vi "SendBuffReceiveCS (SubVI).vi"(8 "error in (no error)":errorcluster, 9 "Array in":u8[](array[numeric]), 10 "ExpectedCheckSum":string, 11 "VISA Refnum in":refnum<visa-resource-name>) -> (0 "error out":errorcluster, 1 "CorrectCheckSum?":bool, 2 "Timeout?":bool, 3 "VISA Refnum out":refnum<visa-resource-name>)   [LabVIEW 2017]
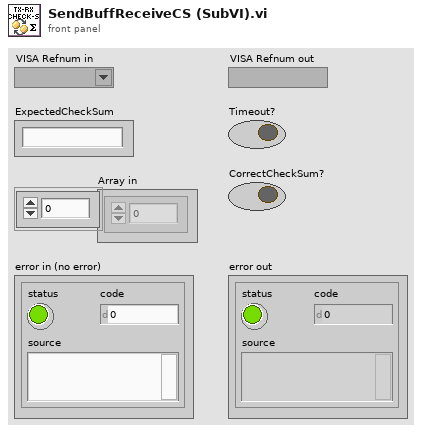
[diagram p1: front panel]
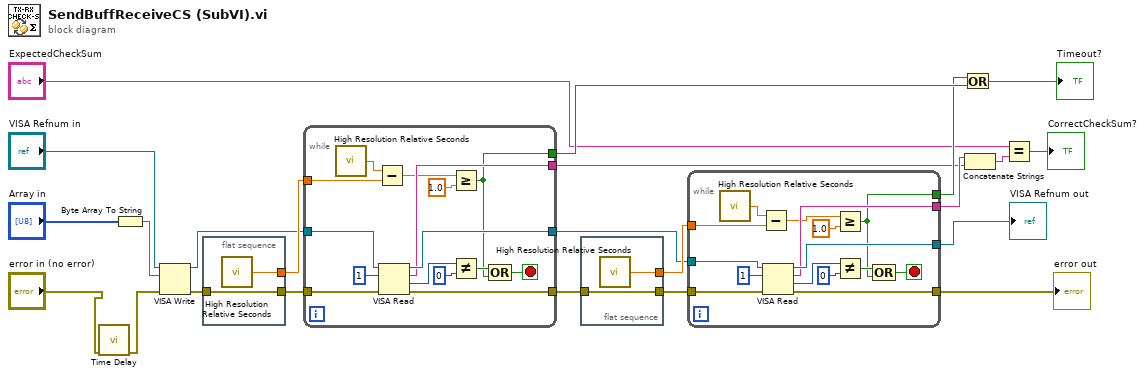
[diagram p0: block diagram]
diagram:
  n1 = call "Time Delay"("error in (no error)"="error in (no error)") -> ("error out"=w1:errorcluster)  [unwired: 10 in]
  n2 = Byte Array To String(unsigned byte array="Array in") -> (string=w23:string)
  n3 = VISA Write(VISA resource name="VISA Refnum in", write buffer=w23, error in (no error)=w1) -> (VISA resource name out=w16:refnum<visa-resource-name>, error out=w17:errorcluster)  [unwired: 1 out]
  n4 = flat-sequence {
    tunnel: [w25] -> w19
    tunnel: w17 -> [w24]
    tunnel: [w24] -> w18
    frame #0 {
      n5 = call <vilib>:"High Resolution Relative Seconds.vi"() -> ("relative seconds"=w25:dbl)
    }
  }
  n6 = while {
    tunnel: w16 -> [w37]
    tunnel: [w38] -> w3
    tunnel: [w39] -> w15
    tunnel: [w32] -> w7
    tunnel: w18 -> [w28]
    tunnel: w19 -> [w27]
    tunnel: [w26] -> w21
    stop <- w34 stop-if-true
    n7 = call <vilib>:"High Resolution Relative Seconds.vi"() -> ("relative seconds"=w29:dbl)
    n8 = Subtract(x=w29, y=w27) -> (x-y=w30:dbl)
    n9 = VISA Read(VISA resource name=w37, byte count=u32 1, error in (no error)=w28) -> (VISA resource name out=w38:refnum<visa-resource-name>, read buffer=w32:string, return count=w33:u32, error out=w39:errorcluster)
    n10 = Greater Or Equal?(x=w30, y=1.0) -> (x >= y?=w26:bool)
    n11 = Not Equal?(x=w33, y=u32 0) -> (x != y?=w35:bool)
    n12 = Compound Arithmetic op=OR(w35, w26) -> (w34:bool)
  }
  n13 = flat-sequence {
    tunnel: w15 -> [w42]
    tunnel: [w42] -> w14
    tunnel: [w41] -> w13
    frame #0 {
      n14 = call <vilib>:"High Resolution Relative Seconds.vi"() -> ("relative seconds"=w41:dbl)
    }
  }
  n15 = while {
    tunnel: w3 -> [w56]
    tunnel: [w53] -> w6
    tunnel: w14 -> [w57]
    tunnel: [w54] -> w5
    tunnel: [w48] -> w8
    tunnel: w13 -> [w44]
    tunnel: [w43] -> w20
    stop <- w49 stop-if-true
    n16 = call <vilib>:"High Resolution Relative Seconds.vi"() -> ("relative seconds"=w47:dbl)
    n17 = Subtract(x=w47, y=w44) -> (x-y=w46:dbl)
    n18 = VISA Read(VISA resource name=w56, byte count=u32 1, error in (no error)=w57) -> (VISA resource name out=w53:refnum<visa-resource-name>, read buffer=w48:string, return count=w50:u32, error out=w54:errorcluster)
    n19 = Greater Or Equal?(x=w46, y=1.0) -> (x >= y?=w43:bool)
    n20 = Not Equal?(x=w50, y=u32 0) -> (x != y?=w52:bool)
    n21 = Compound Arithmetic op=OR(w52, w43) -> (w49:bool)
  }
  "VISA Refnum out" <- w6
  "error out" <- w5
  n22 = Or(x=w20, y=w21) -> (x .or. y?=→"Timeout?":bool)
  n23 = Concatenate Strings(w8, w7) -> (w9:string)
  n24 = Equal?(x="ExpectedCheckSum", y=w9) -> (x = y?=→"CorrectCheckSum?":bool)
